vi "Background Level Global.vi"() -> ()   [LabVIEW 2017, in "DAQ.lvlib"]
uses:
  DAQ.lvlib
panel:
  in  "DAQ Background Level (V)":dbl
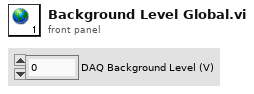
[diagram p1: front panel]
diagram:
